vi "FeedForward.vi"(0 "opinons":dbl[](array[numeric]), 1 "inputs":dbl[][](array[numeric])) -> (8 "output":dbl[](array[numeric]), 9 "Hidden Layer Weights":cluster{"thetas":dbl[], "offset":dbl}[](array[cluster]), 10 "Output Layer Weights":cluster{"thetas":dbl[], "offset":dbl}[](array[cluster]))   [LabVIEW 2014]
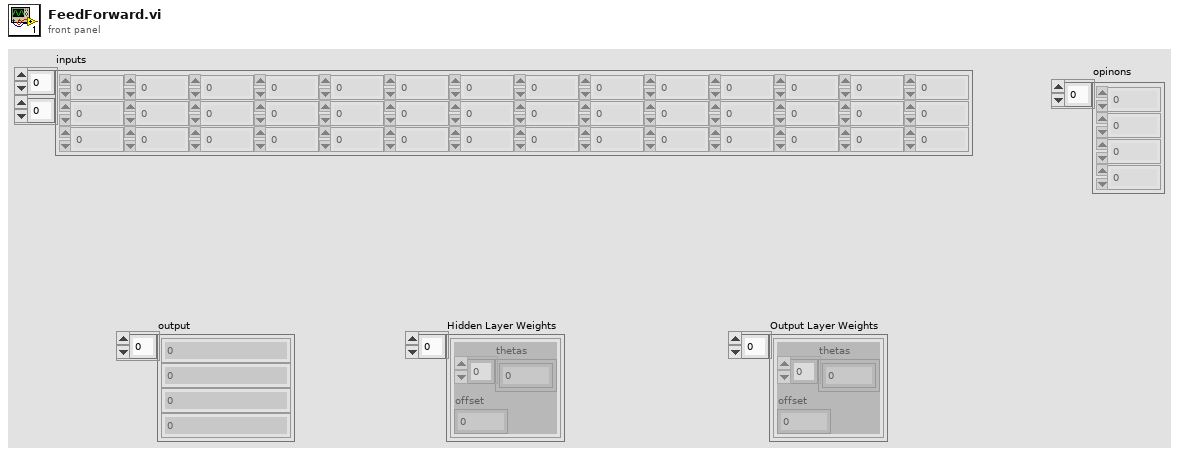
[diagram p1: front panel]
types:
  T1 = enum16{"Single Node", "1 Hidden Level", "2 Hidden Levels"}
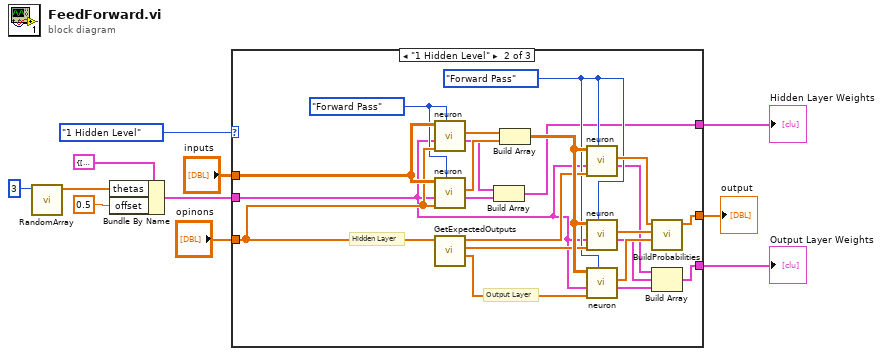
[diagram p0: block diagram]
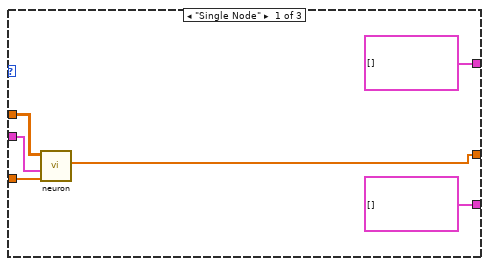
[diagram p2: hidden frame]
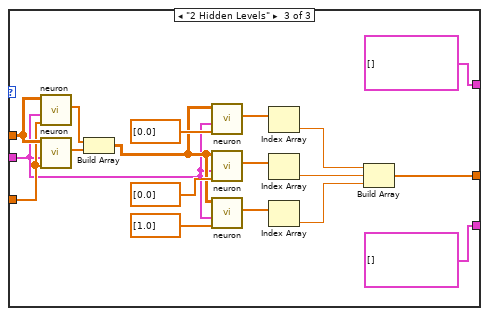
[diagram p3: hidden frame]
diagram:
  n1 = call "RandomArray.vi"("Numeric"=3) -> ("Array"=w5:dbl[])  [unwired: 10 in]
  n2 = Bundle By Name(cluster=cluster{"thetas":dbl[], "offset":dbl} {"thetas"=[], "offset"=0.0} ("Weights"), "thetas"=w5, "offset"=0.5) -> (w3:cluster{"thetas":dbl[], "offset":dbl})
  n3 = case shown="\"1 Hidden Level\"" T1."1 Hidden Level" {
    tunnel: [w15 w32 w44] -> w11
    tunnel: "inputs" -> [w17 w38 w56]
    tunnel: "opinons" -> [w16 w31 w43]
    tunnel: w3 -> [w14 w18 w42]
    tunnel: [cluster{"thetas":dbl[], "offset":dbl}[] [] w24 cluster{"thetas":dbl[], "offset":dbl}[] []] -> w2
    tunnel: [cluster{"thetas":dbl[], "offset":dbl}[] [] w19 cluster{"thetas":dbl[], "offset":dbl}[] []] -> w1
    frame "Single Node" {
      n4 = call "neuron.vi"("opinons"=w16, "Weights"=w14, "inputs"=w17) -> ("output"=w15:dbl[])  [unwired: 7 in, 1 out]
    }
    frame "1 Hidden Level" {
      w26 = enum16{"Forward Pass"}."Forward Pass" ("Enum")
      w27 = enum16{"Forward Pass"}."Forward Pass" ("Enum")
      # "Output Layer"
      # "Hidden Layer"
      n5 = call "neuron.vi"("Enum"=w26, "opinons"=w31, "Weights"=w18, "inputs"=w38) -> ("updated weights"=w25:cluster{"thetas":dbl[], "offset":dbl}, "output"=w37:dbl[])  [unwired: 6 in]
      n6 = call "neuron.vi"("Enum"=w26, "opinons"=w31, "Weights"=w18, "inputs"=w38) -> ("updated weights"=w23:cluster{"thetas":dbl[], "offset":dbl}, "output"=w39:dbl[])  [unwired: 6 in]
      n7 = call "GetExpectedOutputs.vi"("opinons"=w31) -> ("z"=w28:dbl[], "y"=w29:dbl[], "x"=w30:dbl[])  [unwired: 8 in]
      n8 = Build Array(w25, w23) -> (w24:cluster{"thetas":dbl[], "offset":dbl}[])
      n9 = Build Array(w37, w39) -> (w36:dbl[][])
      n10 = call "neuron.vi"("Enum"=w27, "opinons"=w30, "Weights"=w18, "inputs"=w36) -> ("updated weights"=w22:cluster{"thetas":dbl[], "offset":dbl}, "output"=w35:dbl[])  [unwired: 6 in]
      n11 = call "neuron.vi"("Enum"=w27, "opinons"=w29, "Weights"=w18, "inputs"=w36) -> ("updated weights"=w21:cluster{"thetas":dbl[], "offset":dbl}, "output"=w34:dbl[])  [unwired: 6 in]
      n12 = call "neuron.vi"("Enum"=w27, "opinons"=w28, "Weights"=w18, "inputs"=w36) -> ("updated weights"=w20:cluster{"thetas":dbl[], "offset":dbl}, "output"=w33:dbl[])  [unwired: 6 in]
      n13 = call "BuildProbabilities.vi"("z"=w33, "y"=w34, "x"=w35) -> ("xyz"=w32:dbl[])  [unwired: 8 in]
      n14 = Build Array(w22, w21, w20) -> (w19:cluster{"thetas":dbl[], "offset":dbl}[])
    }
    frame "2 Hidden Levels" {
      n15 = call "neuron.vi"("opinons"=w43, "Weights"=w42, "inputs"=w56) -> ("output"=w55:dbl[])  [unwired: 7 in, 1 out]
      n16 = call "neuron.vi"("opinons"=w43, "Weights"=w42, "inputs"=w56) -> ("output"=w57:dbl[])  [unwired: 7 in, 1 out]
      n17 = Build Array(w55, w57) -> (w51:dbl[][])
      n18 = call "neuron.vi"("opinons"=dbl[] [0.0], "Weights"=w42, "inputs"=w51) -> ("output"=w50:dbl[])  [unwired: 7 in, 1 out]
      n19 = call "neuron.vi"("opinons"=dbl[] [0.0], "Weights"=w42, "inputs"=w51) -> ("output"=w49:dbl[])  [unwired: 7 in, 1 out]
      n20 = call "neuron.vi"("opinons"=dbl[] [1.0], "Weights"=w42, "inputs"=w51) -> ("output"=w48:dbl[])  [unwired: 7 in, 1 out]
      n21 = Index Array(array=w50) -> (element=w45:dbl)  [unwired: 1 in]
      n22 = Index Array(array=w49) -> (element=w46:dbl)  [unwired: 1 in]
      n23 = Index Array(array=w48) -> (element=w47:dbl)  [unwired: 1 in]
      n24 = Build Array(w45, w46, w47) -> (w44:dbl[])
    }
  }
  "output" <- w11
  "Hidden Layer Weights" <- w2
  "Output Layer Weights" <- w1
